vi "Initialise.vi"(8 "error in (no error)":errorcluster, 11 "Renderer":u32) -> (0 "error out":errorcluster, 3 "Galaxy out":refnum<class "Galaxy.lvclass">)   [LabVIEW 2021, in "Galaxy.lvclass"]
uses:
  Galaxy.lvclass
  Re-use Libraries/Vector 2D/Vector 2D.lvclass/Vector 2D.ctl
  Star.ctl
  Re-use Libraries/Vector 2D/Vector 2D.lvclass
  Galaxy.lvclass/Galaxy.ctl
  <vilib>/numeric/Random Number (Range) I64.vi
  <vilib>/numeric/Random Number (Range) DBL.vi
  <vilib>/numeric/sub_Random U32.vi
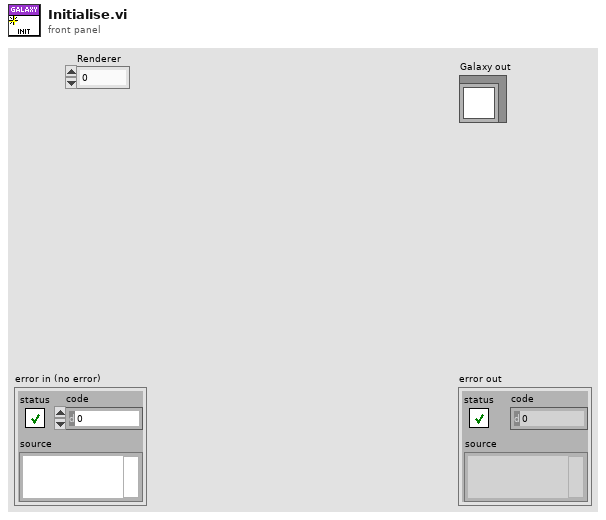
[diagram p1: front panel]
types:
  T1 = typedef "Constants.ctl" = cluster{"Colours":cluster{"OK":u32, "Warning":u32, "Error":u32, "Red":u32, "Green":u32, "Blue":u32, "Yellow":u32}, "System":cluster{"Target Frames Second":dbl, "World Size":T2, "Window Size":T2, "Battle Area Size":T2, "Sidebar Width":sgl, "SC2 Frame Rate [Seconds/Frame]":sgl, "Sidebar Player 2 Y Offset":sgl, "Windows Size V2":refnum<class "Vector 2D.lvclass">, "World Size V2":refnum<class "Vector 2D.lvclass">, "Battle Area Size V2":refnum<class "Vector 2D.lvclass">}, "Game":cluster{"Maximum Asteroids":i32, "Max Energy":i32, "Max Crew":i32, "Maximum Stars":i32}}
  T2 = typedef "SDL2 Utility.lvlib/Point (I32).ctl" = cluster{"x":i32, "y":i32}
  T3 = typedef "Galaxy.lvclass/Star.ctl" = cluster{"Position":refnum<class "Vector 2D.lvclass">, "Texture Index":i32}
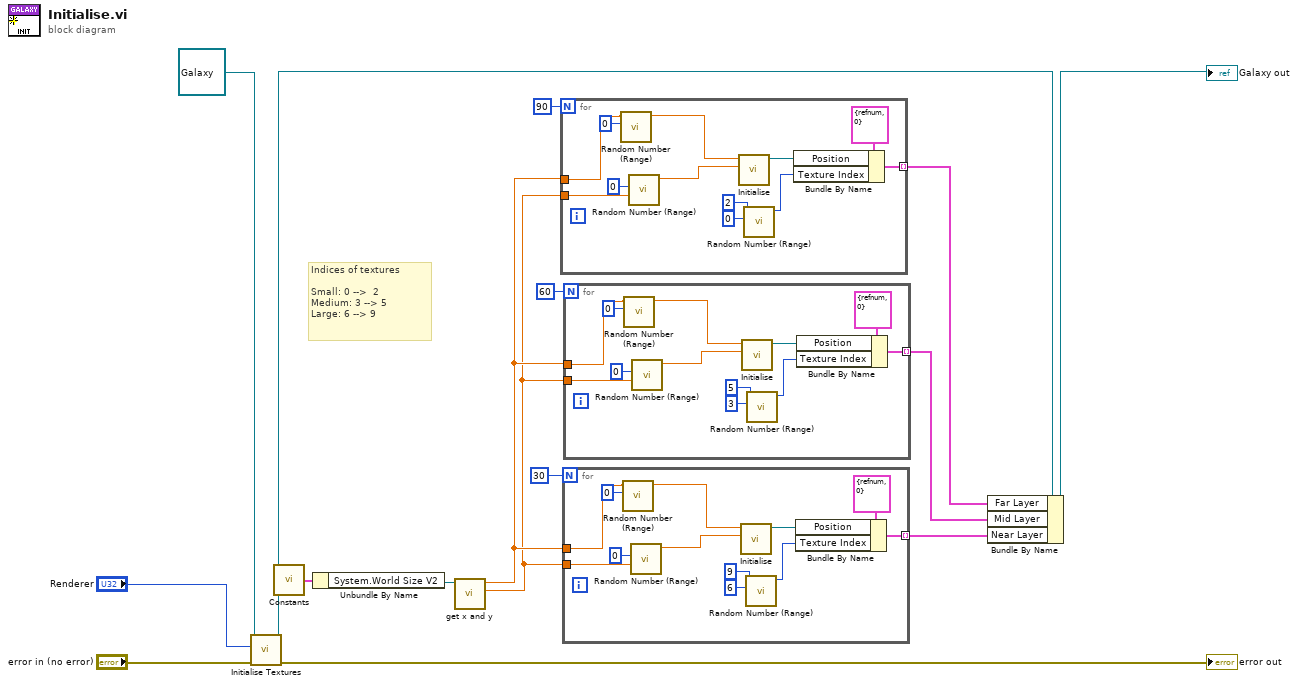
[diagram p0: block diagram]
diagram:
  # "Indices of textures\n\nSmall: 0 -->  2\nMedium: 3 --> 5\nLarge: 6 --> 9"
  n1 = call "Initialise Textures.vi"("error in (no error)"="error in (no error)", "Renderer"="Renderer", "Galaxy in"=refnum<class "Galaxy.lvclass"> refnum) -> ("error out"=→"error out":errorcluster, "Galaxy out"=w12:refnum<class "Galaxy.lvclass">)  [unwired: 7 in]
  n2 = call "Constants.vi"() -> ("Constants"=w8:T1)
  n3 = Unbundle By Name(w8) -> ("System.World Size V2"=w3:refnum<class "Vector 2D.lvclass">)
  n4 = call "get x and y.vi"("Vector 2D in"=w3) -> ("y"=w1:sgl, "x"=w2:sgl)  [unwired: 9 in]
  n5 = for {
    N: 90 -> [_]
    tunnel: [w27] -> w4 mode=indexing
    tunnel: w2 -> [w26]
    tunnel: w1 -> [w21]
    n6 = call-poly <vilib>:"Random Number (Range).vi"("lower bound (0)"=i64 0 ("lower bound (-100)"), "upper bound (100)"=w26) -> ("number"=w23:dbl)  [unwired: 9 in]
    n7 = call-poly <vilib>:"Random Number (Range).vi"("lower bound (0)"=i64 0 ("lower bound (-100)"), "upper bound (100)"=w21) -> ("number"=w20:dbl)  [unwired: 9 in]
    n8 = call "Initialise.vi"("y"=w20, "x"=w23) -> ("Vector 2D out"=w24:refnum<class "Vector 2D.lvclass">)  [unwired: 9 in]
    n9 = call-poly <vilib>:"Random Number (Range).vi"("lower bound (-100)"=i64 0, "upper bound (100)"=i64 2) -> ("number"=w17:i64)  [unwired: 9 in]
    n10 = Bundle By Name(cluster=T3 {"Position"=refnum, "Texture Index"=0} ("Star"), "Position"=w24, "Texture Index"=w17) -> (w27:T3)
  }
  n11 = for {
    N: 30 -> [_]
    tunnel: [w39] -> w9 mode=indexing
    tunnel: w2 -> [w38]
    tunnel: w1 -> [w33]
    n12 = call-poly <vilib>:"Random Number (Range).vi"("lower bound (0)"=i64 0 ("lower bound (-100)"), "upper bound (100)"=w38) -> ("number"=w35:dbl)  [unwired: 9 in]
    n13 = call-poly <vilib>:"Random Number (Range).vi"("lower bound (0)"=i64 0 ("lower bound (-100)"), "upper bound (100)"=w33) -> ("number"=w32:dbl)  [unwired: 9 in]
    n14 = call "Initialise.vi"("y"=w32, "x"=w35) -> ("Vector 2D out"=w36:refnum<class "Vector 2D.lvclass">)  [unwired: 9 in]
    n15 = call-poly <vilib>:"Random Number (Range).vi"("lower bound (-100)"=i64 6, "upper bound (100)"=i64 9) -> ("number"=w29:i64)  [unwired: 9 in]
    n16 = Bundle By Name(cluster=T3 {"Position"=refnum, "Texture Index"=0} ("Star"), "Position"=w36, "Texture Index"=w29) -> (w39:T3)
  }
  n17 = for {
    N: 60 -> [_]
    tunnel: [w51] -> w6 mode=indexing
    tunnel: w2 -> [w50]
    tunnel: w1 -> [w45]
    n18 = call-poly <vilib>:"Random Number (Range).vi"("lower bound (0)"=i64 0 ("lower bound (-100)"), "upper bound (100)"=w50) -> ("number"=w47:dbl)  [unwired: 9 in]
    n19 = call-poly <vilib>:"Random Number (Range).vi"("lower bound (0)"=i64 0 ("lower bound (-100)"), "upper bound (100)"=w45) -> ("number"=w44:dbl)  [unwired: 9 in]
    n20 = call "Initialise.vi"("y"=w44, "x"=w47) -> ("Vector 2D out"=w48:refnum<class "Vector 2D.lvclass">)  [unwired: 9 in]
    n21 = call-poly <vilib>:"Random Number (Range).vi"("lower bound (-100)"=i64 3, "upper bound (100)"=i64 5) -> ("number"=w41:i64)  [unwired: 9 in]
    n22 = Bundle By Name(cluster=T3 {"Position"=refnum, "Texture Index"=0} ("Star"), "Position"=w48, "Texture Index"=w41) -> (w51:T3)
  }
  n23 = Bundle By Name(cluster=w12, "Far Layer"=w4, "Mid Layer"=w6, "Near Layer"=w9) -> (→"Galaxy out":refnum<class "Galaxy.lvclass">)
